vi "AB_Engine_RESTful_Build_App_Name.vi"(11 "service name":string) -> (3 "app name":string)   [LabVIEW 2020]
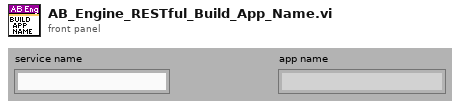
[diagram p1: front panel]
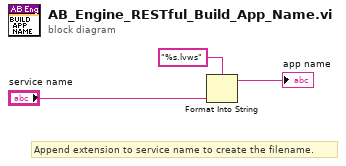
[diagram p0: block diagram]
diagram:
  # "Append extension to service name to create the filename."
  n1 = Format Into String(format string="%s.lvws", "service name") -> (resulting string=→"app name":string)  [unwired: 2 in, 1 out]
